vi "Pre Launch Init.vi"(11 "Form Server in":refnum<class "Form Server.lvclass">) -> (0 "error out":errorcluster, 3 "Form Server out":refnum<class "Form Server.lvclass">)   [LabVIEW 2020, in "Form Server.lvlib" / "Form Server.lvclass"]
doc: "(<B>Filename</B>: Actor Framework.lvlib:Actor.lvclass:Pre Launch Init.vi)\n\nDefines behavior that occurs after the Launch Nested Actor method is invoked but before the actor's Actor Core method begins running.\n\nBy default, this method does nothing. A descendant class may override it to define behavior."
uses:
  Form Server.lvclass
  <vilib>/MGI/Monitored Actor/Monitored Actor/Monitored Actor/Monitored Actor.lvclass
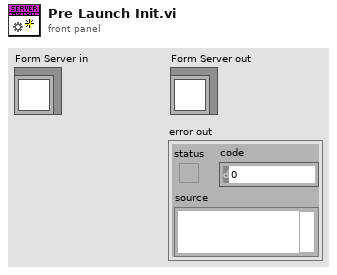
[diagram p1: front panel]
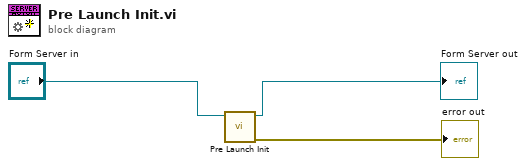
[diagram p0: block diagram]
diagram:
  n1 = call-parent "Pre Launch Init.vi"("Monitored Actor in"="Form Server in") -> ("error out"=→"error out":errorcluster, "Monitored Actor out"=→"Form Server out":refnum<class "Form Server.lvclass">)  [unwired: 9 in]
